vi "Get frame sequence.vi"(7 "Signal Channel":enum16{"Red", "Green"}(ring), 8 "Error In":errorcluster, 10 "AOL Z values":i32[](array[numeric]), 11 "Motor Z values":i32[](array[numeric])) -> (0 "Error Out":errorcluster, 3 "Array":T1[](array[plugin-control]))   [LabVIEW 2020]
uses:
  Peripherals Control/XYZ Stage/Typedefs/XYZ stage data.ctl
  Peripherals Control/XYZ Stage/Typedefs/XYZ stage states.ctl
  Peripherals Control/XYZ Stage/Typedefs/XYZ channel ring.ctl
  Typedefs/Top level VI states.ctl
  Global Variables/gl_UI Ctrl Refs.vi
  Global Variables/gl_Images.vi
  <vilib>/vision/NI_Vision_Development_Module.lvlib
panel:
  in  "Delay":u32=2000
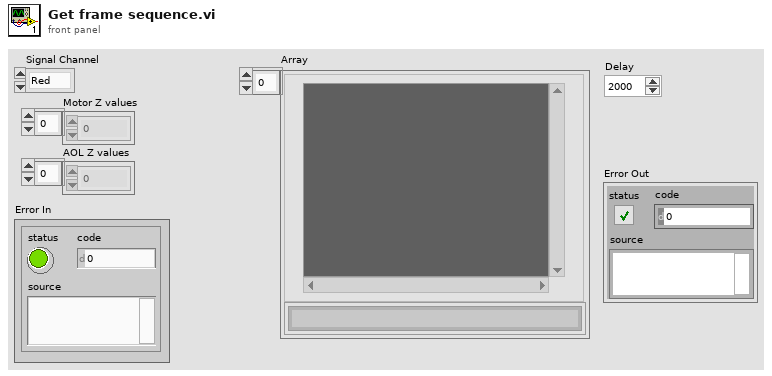
[diagram p1: front panel]
types:
  T1 = typedef "IMAQ Image.ctl" = refnum<image>
  T2 = typedef "UI ctrl refs cluster.ctl" = cluster{"Top level VI path":path, "Top level VI ref":refnum<vi>, "User menu ref":refnum<k9>, "Sub Panel control":refnum<vi>, "Imaging Param Tab":refnum<vi>, "Occurrence-Start drivers":refnum<k4>, "Occurrence-Speed logging initialised":refnum<k4>, "Occurrence-XYZ stage initialised":refnum<k4>, "Exit button":refnum<vi>, "Status ind":refnum<vi>, "Set as origin":refnum<vi>, "Speed Logging":refnum<vi>, "Time Lapse":refnum<vi>, "Live Imaging":refnum<vi>, "AOL Z Stack":refnum<vi>, "Motor Z Stack":refnum<vi>, "Funct Acq button":refnum<vi>, "Hard Shutter":refnum<vi>, "Virtual Shutter":refnum<vi>, "Laser Power":refnum<vi>, "AOL Mode":refnum<vi>, "Frame Size":refnum<vi>, "Field of View":refnum<vi>, "Dwell Time":refnum<vi>, "Zoom":refnum<vi>, "AOL Z":refnum<vi>, "Objective":refnum<vi>, "Axis":refnum<vi>, "Paths & Names":refnum<vi>, "Experiment folder path (ind.)":refnum<vi>, "Last State (Ind.)":refnum<vi>, "Averages":refnum<vi>, "Angle (degrees)":refnum<vi>, "X centre":refnum<vi>, "Y centre":refnum<vi>, "Plane Mode":refnum<vi>, "# Planes":refnum<vi>, "Z Start":refnum<vi>, "Z Stop":refnum<vi>, "Z Step":refnum<vi>, "PMT 1":refnum<vi>, "PMT 2":refnum<vi>, "Stage XYZ Position":refnum<vi>, "Pockels@Z Start":refnum<vi>, "Pockels@Z Stop":refnum<vi>, "Obtain Z Start":refnum<vi>, "Obtain Z Stop":refnum<vi>, "Live stim.trig.period":refnum<vi>, "Live stim.trig.enable":refnum<vi>, "Movement Correction":refnum<vi>, "Load Reference Image":refnum<vi>, "XY Stage Move":refnum<vi>, "MovCor Cluster":refnum<vi>, "RefDAQParam":refnum<vi>, "Funct. Acq. Pockels Modulation":refnum<vi>, "Ref Laser Power":refnum<vi>, "Enable Video Recording":refnum<vi>, "Video Record-Live Imaging":refnum<vi>, "Video Record-Funct acq":refnum<vi>, "Reference Source":refnum<vi>, "AOL Z-stack Chirps Ready (ind)":refnum<vi>, "Target time between mov.cor. ref triggers (ms)":refnum<vi>, "Funct. Acq. Ref frame save":refnum<vi>, "Tracking button":refnum<vi>, "Show ref plots window":refnum<vi>, "Center freq ind (nm)":refnum<vi>, "Pickup mode (ind)":refnum<vi>, "Logging queue (ind)":refnum<vi>, "Back aperture power (ind.)":refnum<vi>, "Power after objective (ind.)":refnum<vi>, "Switch user":refnum<vi>, "Ls1 Conn. Status":refnum<vi>, "Ls1Tuning Status":refnum<vi>, "Ls1 Faults":refnum<vi>, "Ls1 Connection":refnum<vi>, "Ls1 Mode":refnum<vi>, "Ls1 POWER [mW]":refnum<vi>, "Ls1Shutter":refnum<vi>, "Ls1 Wavelength":refnum<vi>, "Ls1 Note":refnum<vi>, "Ls1 Confirm Wav":refnum<vi>, "Ls1 PreChrp Prism1":refnum<vi>, "Ls1 PreChrp Prism2":refnum<vi>, "Ls1 wav top Ind":refnum<vi>, "Ls1 power top Ind":refnum<vi>, "Ls1 Pump peak Hold":refnum<vi>, "Ls1 Status Ind":refnum<vi>, "Ls1 wav cancel":refnum<vi>, "Experiment Type":refnum<vi>, "Biology Information":refnum<vi>, "Camera recording status":refnum<vi>, "Optimise Obj. Pos.":refnum<vi>}
  T3 = typedef "XYZ stage states.ctl" = enum16{"Dequeue", "Initialize", "Read Position", "Read Speed Setting", "Move", "Set Max Speed", "Reset Axis", "Stop all movement"}
  T4 = typedef "XYZ channel ring.ctl" = string
  T5 = typedef "XYZ stage data.ctl" = cluster{"Command":T3, "Channel":T4, "X":sgl, "Y":sgl, "Z":sgl, "Speed":i32, "Zero":bool, "Use acknowledgement?":bool}
  T6 = typedef "Top level VI states.ctl" = enum16{"None", "Initialise UI", "<STACK PROTOCOL STATES>", "AOL Zstack-START", "AOL Zstack-STOP", "Motor Zstack-START", "Motor Zstack-STOP", "Parameter Sweep-START", "Parameter Sweep-STOP", "<ACQUISITION PROTOCOL STATES> ", "Functional Acquisition-START", "Functional Acquisition-STOP", "Single Plane Acquisition-START", "Single Plane Acquisition-STOP", "Volume Acquisition-START", "Volume Acquisition-STOP", "<LIVE IMAGING PROTOCOL STATES>", "Live Imaging-START", "Live Imaging-STOP", "Live Plane Imaging-START", "Live Plane Imaging-STOP", "Live Volume Imaging-START", "Live Volume Imaging-STOP", "<MOVEMENT CORRECTION PROTOCOL STATES>", "EXIT"}
  T7 = typedef "Image Type" = u32
  T8 = typedef "AOL_Globals.ctl" = cluster{"Imaging Protocol":T9, "Number of POI":u16, "Number of Miniscans":u16, "Number of Trials":u16, "Number of Cycles ":u64, "# Averaged Frames":u16, "Laser power (%)":u8, "Pockels (V)":dbl, "Acquisition Length (sec)":dbl, "Fill time (us)":dbl, "POI Dwell time (us)":dbl, "Miniscan Dwell time per pixel (us)":dbl, "PMT 1":dbl, "PMT 2":dbl, "Back Apperture (mA)":dbl, "Frame Size":T10, "Center Frequency":dbl, "Field of View (um)":dbl, "Field of View (norm)":dbl, "DwellTime (us)":dbl, "Ref Dwell Time (us)":dbl, "Wavelength (nm)":dbl, "Zoom":dbl, "AOL Z":dbl, "AOL Mode":T11, "GridXY":dbl, "GridZ":dbl, "TriggerPeriod (sec)":dbl, "Number of Pixels in Miniscan":u16, "Experiment folder path":path, "X centre":dbl, "Y centre":dbl, "Angle (degrees)":dbl, "Angle Xs (degrees)":dbl, "Angle Ys (degrees)":dbl, "Plane Mode":T12, "Threshold":u16[], "Regenerate Chirps":bool, "Rectangle ROI length (pixels)":u16, "Rectangle ROI height (pixels)":u16, "AOD fill":u16, "StartupDelay":i32, "Samples Wait after Trigger":u16, "Slip Cycle":u32, "Add Cycle":bool, "Functional Mode":T13, "Z Start":dbl, "Z Stop":dbl, "# Planes":i32, "Total Pixels":i32, "Variable Miniscan Pixels":u16[], "Use Variable Length":bool, "Use Variable Resolution":bool, "Laser power (%) at Z Start":u8, "Laser power (%) at Z Stop":u8, "Ref Z Step":i8}
  T9 = typedef "Imaging Protocols enum.ctl" = enum16{"AOL Z-Stack", "Motor Z Stack", "Parameter Sweep", "Functional Acquisition", "Single Plane Acquisition", "Volume Acquisition", "Live Imaging", "Live Plane Imaging", "Live Volume Imaging"}
  T10 = typedef "Frame Size.ctl" = u16
  T11 = typedef "AOL modes.ctl" = enum16{"Raster", "Structural", "Pointing", "Mini Scan", "Alignment"}
  T12 = typedef "Plane Mode.ctl" = u16
  T13 = typedef "Functional Mode.ctl" = enum16{"Point", "Line", "Patch", "Plane", "Volume"}
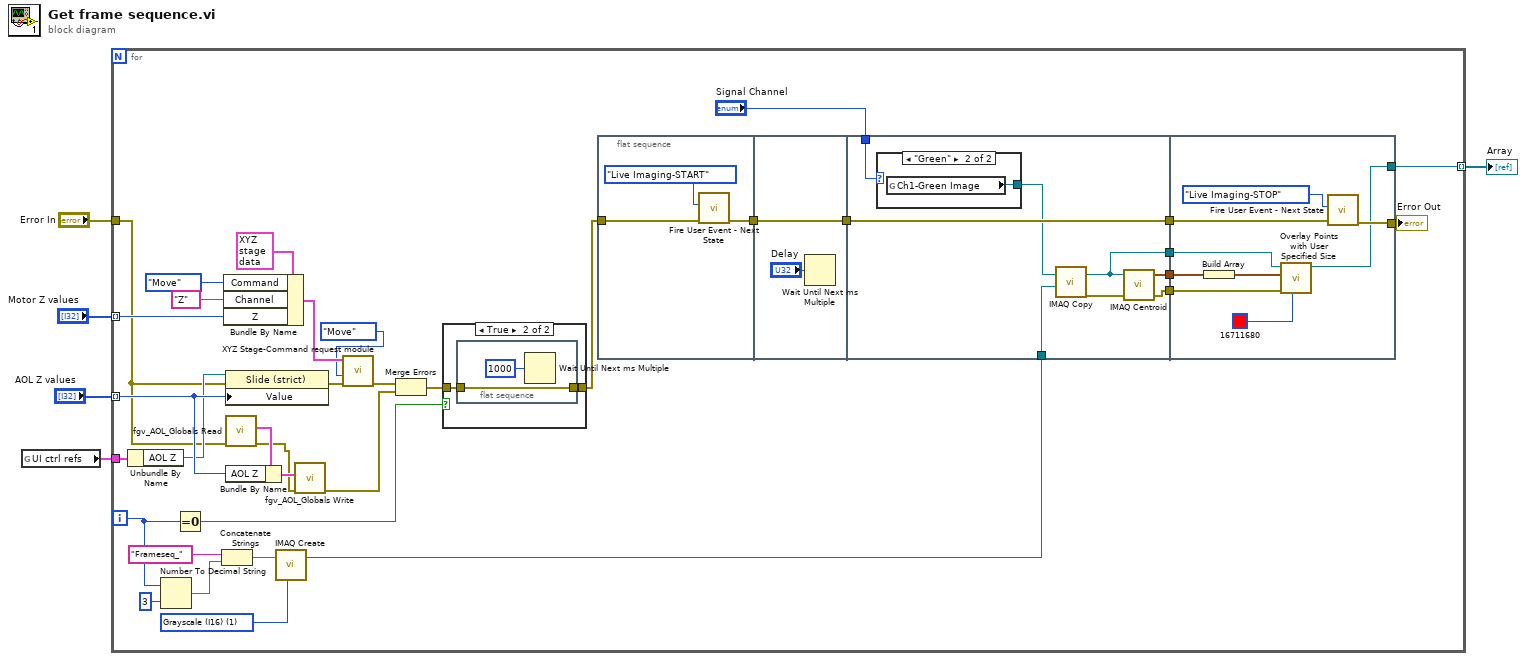
[diagram p0: block diagram]
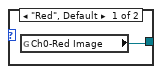
[diagram p3: hidden frame]
diagram:
  n1 = global read "gl_UI Ctrl Refs.vi" "UI ctrl refs"() -> (w1:T2)
  n2 = for {
    tunnel: "Error In" -> [w22]
    tunnel: [w35] -> w4 mode=indexing
    tunnel: "Motor Z values" -> [w27] mode=indexing
    tunnel: "AOL Z values" -> [w26] mode=indexing
    tunnel: w1 -> [w25]
    i -> [w7]
    w14 = T7 1 items=["Grayscale (U8)", "Grayscale (I16)", "Grayscale (SGL)", "Complex (CSG)", "RGB (U32)", "HSL (U32)", "RGB (U64)", "Grayscale (U16)"] ("Image Type")
    n3 = Unbundle By Name(w25) -> ("AOL Z"=w24:refnum<vi>)
    n4 = Number To Decimal String(number=w7, width (-)=i16 3) -> (decimal integer string=w16:string)
    n5 = Equal To 0?(x=w7) -> (x = 0?=w6:bool)
    n6 = Concatenate Strings("Frameseq_", w16) -> (w15:string)
    n7 = Bundle By Name(cluster=T5 {"Command"=enum."Initialize", "Channel"="Z", "X"=0.0, "Y"=0.0, "Z"=0.0, "Speed"=0, "Zero"=FALSE, "Use acknowledgement?"=TRUE} ("XYZ Stage data to queue"), "Command"=XYZ_stage_states."Move", "Channel"=T4 "Z", "Z"=w27) -> (w32:T5)
    n8 = property class="Slide (strict)"(reference=w24, error in=w22, "Value"=w26) -> (error out=w31:errorcluster)  [unwired: 1 out]
    n9 = call "fgv_AOL_Globals Read.vi"("error in (no error)"=w22) -> ("error out"=w21:errorcluster, "AOL_Globals"=w33:T8)  [unwired: 8 in, 1 out]
    n10 = Bundle By Name(cluster=w33, "AOL Z"=w26) -> (w34:T8)
    n11 = call "IMAQ Create"("Image Name"=w15, "Image Type"=w14) -> ("New Image"=w13:T1)  [unwired: 3 in, 1 out]
    n12 = call "fgv_AOL_Globals Write.vi"("error in (no error)"=w21, "AOL_Globals"=w34) -> ("error out"=w19:errorcluster)  [unwired: 9 in]
    n13 = call "XYZ Stage-Command request module.vi"("error in"=w31, "Command"=XYZ_stage_states."Move", "XYZ Stage data to queue"=w32) -> ("error out"=w20:errorcluster)  [unwired: 4 in, 4 out]
    n14 = Merge Errors(w20, w19) -> (w9:errorcluster)
    n15 = case shown="True" w6 {
      tunnel: w9 -> [w41 w43]
      tunnel: [w41 w42] -> w8
      frame False {
      }
      frame True {
        n16 = flat-sequence {
          tunnel: w43 -> [w45]
          tunnel: [w45] -> w42
          frame #0 {
            n17 = Wait Until Next ms Multiple(millisecond multiple=u32 1000) -> ()  [unwired: 1 out]
          }
        }
      }
    }
    n18 = flat-sequence {
      tunnel: w8 -> [w47]
      tunnel: [w46] -> w11
      tunnel: w11 -> [w50]
      tunnel: [w50] -> w10
      tunnel: w10 -> [w58]
      tunnel: [w58] -> w40
      tunnel: "Signal Channel" -> [w57]
      tunnel: [w56] -> w39
      tunnel: [w54] -> w38
      tunnel: w13 -> [w53]
      tunnel: [w51] -> w12
      tunnel: w40 -> [w68]
      tunnel: [w67] -> w37
      tunnel: [w62] -> w35
      tunnel: w39 -> [w65]
      tunnel: w38 -> [w66]
      tunnel: w12 -> [w61]
      frame #0 {
        n19 = call "Fire User Event - Next State.vi"("Error In"=w47, "\"UI Handler loop\" case to execute"=Top_level_VI_states."Live Imaging-START" ("\"UI Handler loop\" case to execute")) -> ("Error Out"=w46:errorcluster)  [unwired: 9 in]
      }
      frame #1 {
        n20 = Wait Until Next ms Multiple(millisecond multiple="Delay") -> ()  [unwired: 1 out]
      }
      frame #2 {
        n21 = case shown="\"Green\"" w57 {
          tunnel: [w59 w60] -> w55
          frame "Red", Default {
            n22 = global read "gl_Images.vi" "Ch0-Red Image"() -> (w59:T1)
          }
          frame "Green" {
            n23 = global read "gl_Images.vi" "Ch1-Green Image"() -> (w60:T1)
          }
        }
        n24 = call "IMAQ Copy"("Image Dst"=w53, "Image Src"=w55) -> ("error out"=w52:errorcluster, "Image Dst Out"=w54:T1)  [unwired: 4 in]
        n25 = call "IMAQ Centroid"("error in (no error)"=w52, "Image"=w54) -> ("error out"=w51:errorcluster, "Centroid"=w56:cluster{"X Centroid":sgl, "Y Centroid":sgl})  [unwired: 2 in]
      }
      frame #3 {
        n26 = Build Array(w65) -> (w64:cluster{"X Centroid":sgl, "Y Centroid":sgl}[])
        n27 = call "Overlay Points with User Specified Size.vi"("Color"=u32 16711680, "error in"=w61, "Points"=w64, "Image In"=w66) -> ("Image Out"=w62:T1)  [unwired: 6 in, 1 out]
        n28 = call "Fire User Event - Next State.vi"("Error In"=w68, "\"UI Handler loop\" case to execute"=Top_level_VI_states."Live Imaging-STOP" ("\"UI Handler loop\" case to execute")) -> ("Error Out"=w67:errorcluster)  [unwired: 9 in]
      }
    }
    "Error Out" <- w37
  }
  "Array" <- w4
